vi "Read ID.vi"(8 "error in (no error)":errorcluster, 11 "PV Data in":refnum<class "PV Data.lvclass">) -> (0 "error out":errorcluster, 2 "ID":string, 3 "PV Data out":refnum<class "PV Data.lvclass">)   [LabVIEW 2020, in "PV Access.lvlib" / "PV Data.lvlib" / "PV Data.lvclass"]
uses:
  PV Data.lvclass
  PV Access.lvlib
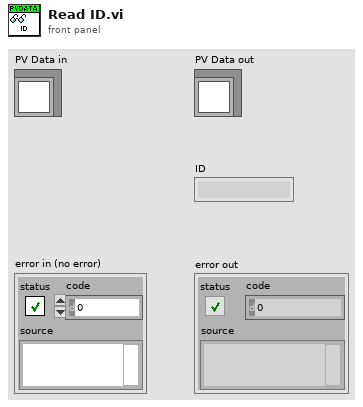
[diagram p1: front panel]
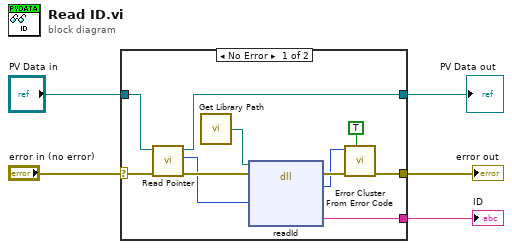
[diagram p0: block diagram]
diagram:
  n1 = case shown="No Error" "error in (no error)" {
    selector: "error in (no error)" -> [w14 w18]
    tunnel: [w9 w18] -> w4
    tunnel: "PV Data in" -> [w13 w17]
    tunnel: [w11 w17] -> w2
    tunnel: [w6 _] -> w1
    frame No Error {
      n2 = call-dynamic "Read Pointer.vi"("error in (no error)"=w14, "Pointer Base in"=w13) -> ("error out"=w15:errorcluster, "Pointer"=w12:i64, "Pointer Base out"=w11:refnum<class "PV Data.lvclass">)  [unwired: 7 in]
      n3 = call "Get Library Path.vi"() -> ("Path"=w16:path)  [unwired: 1 in]
      n4 = dll-call lib="?" fn="readId"(path in=w16, error in=w15, "value"=w12) -> (error out=w10:errorcluster, "err_code"=w7:i32, "ID"=w6:string)  [unwired: 3 in, 1 out]
      n5 = call <vilib>:"Error Cluster From Error Code.vi"("show call chain? (False)"=TRUE, "error in (no error)"=w10, "error code (0)"=w7) -> ("error out"=w9:errorcluster)  [unwired: 6 in]
    }
    frame Error {
    }
  }
  "error out" <- w4
  "PV Data out" <- w2
  "ID" <- w1
